vi "PCU_Cal_All_SOP_Parametar.vi"(8 "error in (no error)":errorcluster, 10 "wave":dbl[](array[numeric]), 11 ".NET Reference in":refnum<k24>) -> (0 "error out":errorcluster, 2 "result out":sgl[][][](array[numeric]), 3 "Reference out":refnum<k24>)   [LabVIEW 2017]
uses:
  D:/test/FULLband-sts/Fullband_Sample/DLL/InstrumentDLL.dll
  DLL/InstrumentDLL.dll
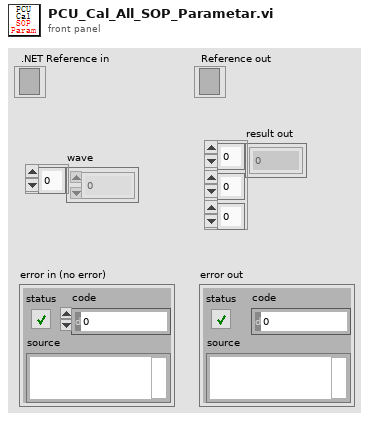
[diagram p1: front panel]
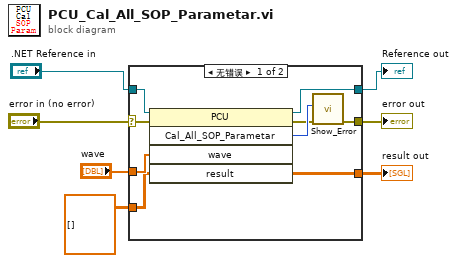
[diagram p0: block diagram]
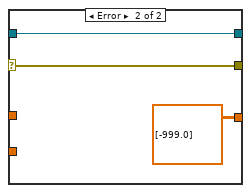
[diagram p2: hidden frame]
diagram:
  n1 = case shown="无错误" "error in (no error)" {
    selector: "error in (no error)" -> [w14 w19]
    tunnel: ".NET Reference in" -> [w16 w18]
    tunnel: [w15 w18] -> w6
    tunnel: [w11 w19] -> w5
    tunnel: [w10 sgl[][][] [[[-999.0]]] ("result")] -> w2
    tunnel: "wave" -> [w9 _]
    tunnel: sgl[][][] [] ("result") -> [w8 _]
    frame No Error {
      n2 = invoke on="调用节点" class="PCU" method="Cal_All_SOP_Parametar"(reference=w16, error in=w14, "wave"=w9, "result"=w8) -> (reference out=w15:refnum<k24>, error out=w12:errorcluster, "Cal_All_SOP_Parametar"=w13:i32, "result"=w10:sgl[][][])  [unwired: 1 in, 1 out]
      n3 = call "Show_Error.vi"("error in (no error)"=w12, "Error"=w13) -> ("error out"=w11:errorcluster)  [unwired: 9 in]
    }
    frame Error {
    }
  }
  "Reference out" <- w6
  "error out" <- w5
  "result out" <- w2
